vi "MNIST.vi"() -> ()   [LabVIEW 2016]
panel:
  out "Output Tensor":sgl[](array[slide]) scale=0.0..1.0
  out "Labels":i32[](array[numeric])=[0, 1, 2, 3, 4, 5, 6, 7, 8, 9]
  out "Path to DLL":path
  out "TensorFlow Ready":bool
  in  "Clear Button":bool
  in  "Stop Button":bool
  out "Picture":picture
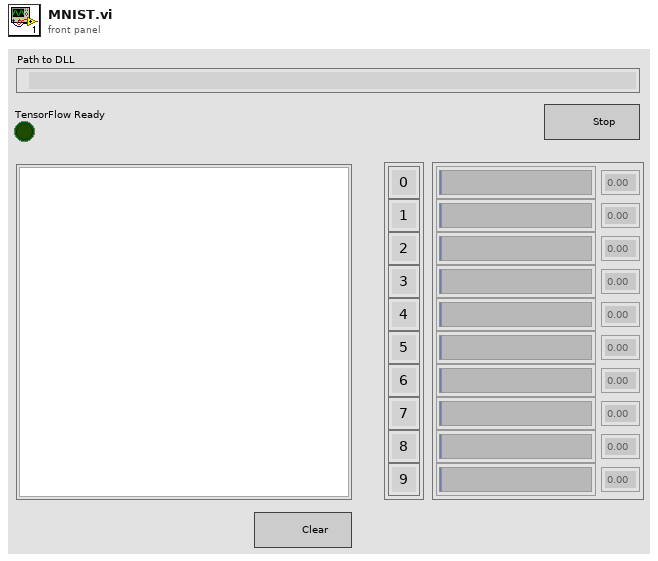
[diagram p1: front panel]
types:
  T1 = typedef "LVPoint32TypeDef.ctl" = cluster{"Horizontal":i32, "Vertical":i32}
  T2 = typedef "LVBoundsTypeDef.ctl" = cluster{"Width":u32, "Height":u32}
  T3 = typedef "LVPositionTypeDef.ctl" = cluster{"Left":i32, "Top":i32}
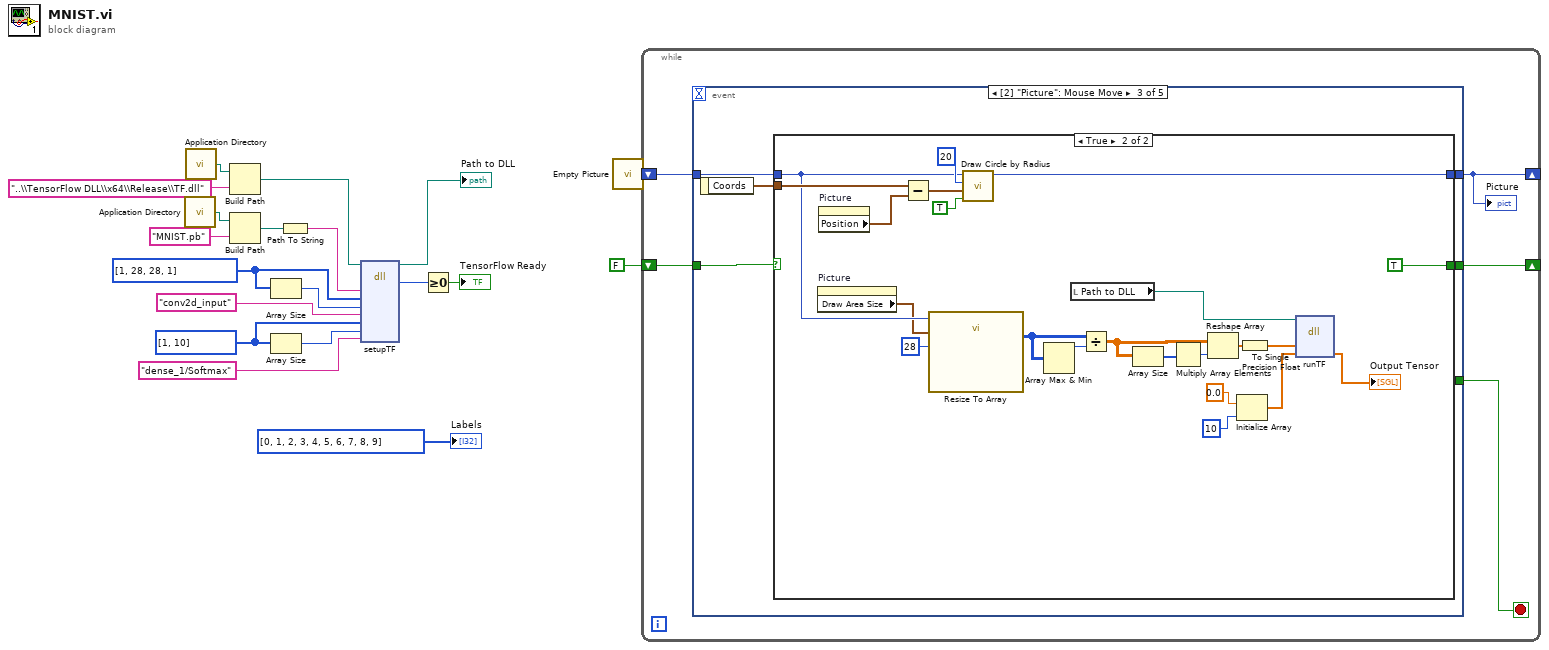
[diagram p0: block diagram]
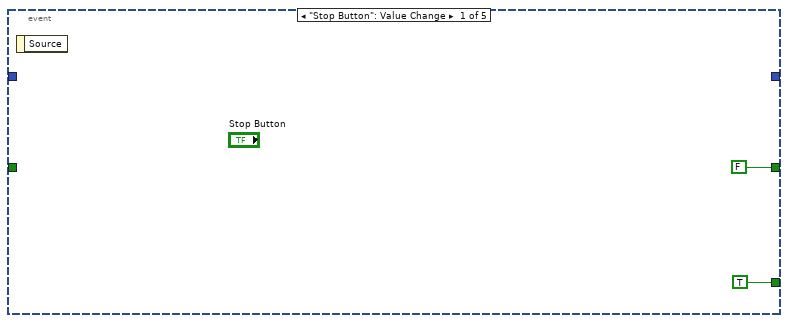
[diagram p2: hidden frame]
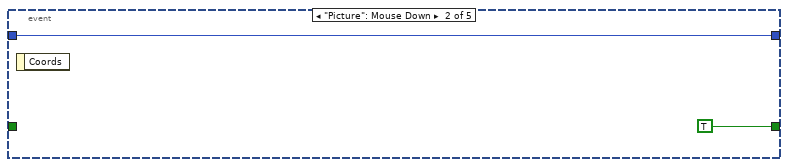
[diagram p3: hidden frame]
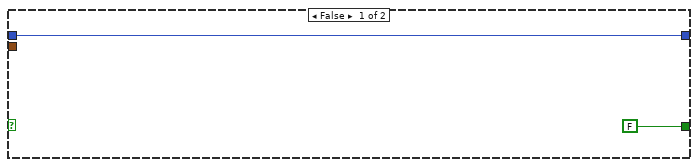
[diagram p4: hidden frame]
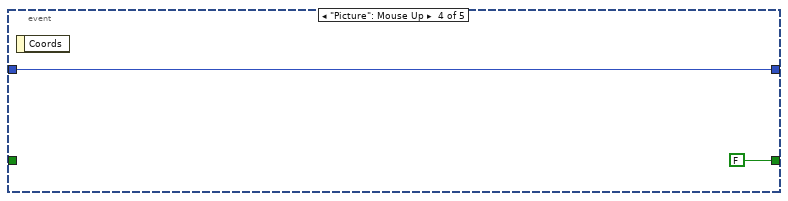
[diagram p5: hidden frame]
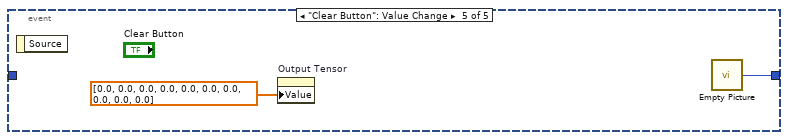
[diagram p6: hidden frame]
diagram:
  w5 = i64[] [1, 28, 28, 1] ("in_shape")
  w1 = i64[] [1, 10] ("in_shape")
  n1 = call <vilib>:"Application Directory.vi"() -> ("Application Directory"=w10:path)
  n2 = call <vilib>:"Application Directory.vi"() -> ("Application Directory"=w14:path)
  n3 = Build Path(base path=w14, name or relative path="..\\TensorFlow DLL\\x64\\Release\\TF.dll" ("string")) -> (appended path=w8:path)
  n4 = Build Path(base path=w10, name or relative path="MNIST.pb" ("string")) -> (appended path=w11:path)
  n5 = Array Size(array=w5) -> (size(s)=w4:i32)
  n6 = Array Size(array=w1) -> (size(s)=w3:i32)
  n7 = Path To String(path=w11) -> (string=w7:string)
  n8 = dll-call lib="?" fn="setupTF"(path in=w8, "file"=w7, "in_shape"=w5, "in_dim"=w4, "in_name"="conv2d_input" ("string"), "out_shape"=w1, "out_dim"=w3, "out_name"="dense_1/Softmax" ("string")) -> (path out=→"Path to DLL":path, "return type"=w13:i32)  [unwired: 9 in, 1 out]
  n9 = Greater Or Equal To 0?(x=w13) -> (x >= 0?=→"TensorFlow Ready":bool)
  n10 = call "Empty Picture"() -> ("empty picture"=w18:picture)
  n11 = while {
    shift-right: [w20] -> _
    shift-left: w18 -> [w23]
    shift-right: [w22] -> _
    shift-left: FALSE -> [w21]
    stop <- w24 stop-if-true
    n12 = event shown="[2] \"Picture\": Mouse Move" {
      selector: _ -> [_ _ _ _ _]
      dyn-events: _ -> [_ _ _ _ _]
      timeout: _ -> [_ _ _ _ _]
      tunnel: [TRUE _ _ _ _] -> w24
      tunnel: w23 -> [_ w27 w30 w58 _]
      tunnel: [_ w27 w29 w58 w61] -> w20
      tunnel: [FALSE TRUE w31 FALSE _] -> w22
      tunnel: w21 -> [_ _ w32 _ _]
      event "Stop Button": Value Change {
        n13 = event-data() -> ()  [unwired: 1 in, 1 out]
      }
      event "Picture": Mouse Down {
        n14 = event-data() -> ()  [unwired: 1 in, 1 out]
      }
      event "Picture": Mouse Move {
        n15 = event-data() -> ("Coords"=w33:T1)  [unwired: 1 in]
        n16 = case shown="True" w32 {
          tunnel: w33 -> [_ w53]
          tunnel: [FALSE TRUE] -> w31
          tunnel: w30 -> [w34 w50]
          tunnel: [w34 w54] -> w29
          frame False {
          }
          frame True {
            n17 = property on="Picture" class="Pict"() -> ("Draw Area Size"=w49:T2)  [unwired: 2 in, 2 out]
            n18 = property on="Picture" class="Pict"() -> ("Position"=w51:T3)  [unwired: 2 in, 2 out]
            n19 = Subtract(x=w53, y=w51) -> (x-y=w52:T1)
            n20 = call "Resize To Array.vi"("New Size (In)"=28, "Draw Area Size (In)"=w49, "Picture (In)"=w50) -> ("Image Array (Out)"=w44:u8[][])  [unwired: 8 in]
            n21 = call <vilib>:"Draw Circle by Radius.vi"("fill?(F)"=TRUE, "pixel center"=w52, "radius"=i16 20, "picture"=w50) -> ("new picture"=w54:picture)  [unwired: 7 in]
            n22 = Array Max & Min(array=w44) -> (max value=w45:u8)  [unwired: 3 out]
            n23 = local read "Path to DLL"() -> (w39:path)
            n24 = Divide(x=w44, y=w45) -> (x/y=w43:dbl[][])
            n25 = Array Size(array=w43) -> (size(s)=w46:i32[])
            n26 = Multiply Array Elements(1:w46) -> (0:w47:i32)
            n27 = Reshape Array(w43, w47) -> (w40:dbl[])
            n28 = Initialize Array(sgl 0.0 ("element"), 10 ("dimension size")) -> (w37:sgl[])
            n29 = To Single Precision Float(number=w40) -> (single precision float=w38:sgl[])
            n30 = dll-call lib="?" fn="runTF"(path in=w39, "input_tensor"=w38, "output_tensor"=w37) -> ("output_tensor"=→"Output Tensor":sgl[])  [unwired: 4 in, 2 out]
          }
        }
      }
      event "Picture": Mouse Up {
        n31 = event-data() -> ()  [unwired: 1 in, 1 out]
      }
      event "Clear Button": Value Change {
        n32 = event-data() -> ()  [unwired: 1 in, 1 out]
        n33 = property on="Output Tensor" class="Arr (strict)"("Value"=sgl[] [0.0, 0.0, 0.0, 0.0, 0.0, 0.0, 0.0, 0.0, 0.0, 0.0]) -> ()  [unwired: 2 in, 2 out]
        n34 = call "Empty Picture"() -> ("empty picture"=w61:picture)
      }
    }
    "Picture" <- w20
  }
  "Labels" <- i32[] [0, 1, 2, 3, 4, 5, 6, 7, 8, 9]
